vi "testPositiveFixInt.vi"(8 "error in (no error)":errorcluster, 11 "TestCase in":refnum<class "MsgPackSerializerTest.lvclass">) -> (0 "error out":errorcluster, 3 "TestCase out":refnum<class "MsgPackSerializerTest.lvclass">)   [LabVIEW 2015, in "MsgPackSerializerTest.lvclass"]
uses:
  MsgPackSerializerTest.lvclass
  MsgPackSerializer/MsgPackSerializer.lvclass
  <vilib>/addons/_JKI Toolkits/VI Tester/TestCase.llb/TestCase.lvclass
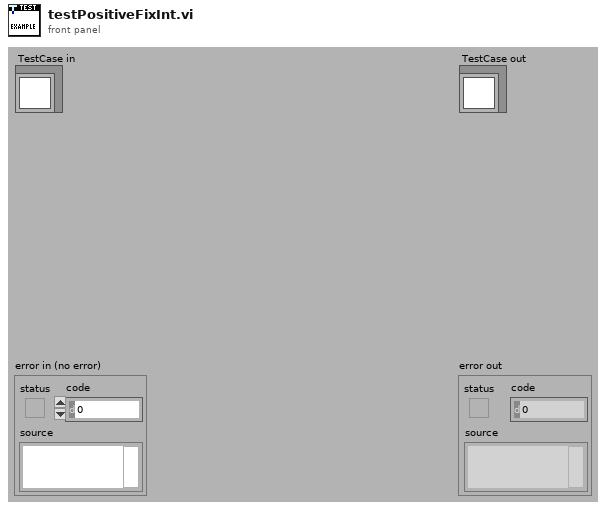
[diagram p1: front panel]
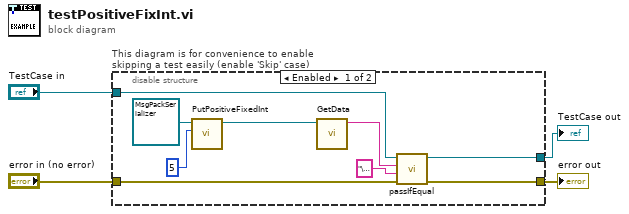
[diagram p0: block diagram]
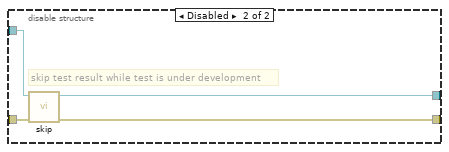
[diagram p2: hidden frame]
diagram:
  n1 = disable-structure "This diagram is for convenience to enable skipping a test easily (enable 'Skip' case)" shown="Enabled" {
    disable-tunnel: "TestCase in" -> [w13 w17]
    disable-tunnel: [w12 w15] -> w1
    disable-tunnel: [w11 w16] -> w3
    disable-tunnel: "error in (no error)" -> [w8 w14]
    frame Enabled {
      n2 = call "PutPositiveFixedInt.vi"("Number"=u8 5, "MsgPackSerializer in"=refnum<class "MsgPackSerializer.lvclass"> refnum ("MsgPackSerializer.lvclass")) -> ("MsgPackSerializer out"=w6:refnum<class "MsgPackSerializer.lvclass">)  [unwired: 8 in, 1 out]
      n3 = call "GetData.vi"("MsgPackSerializer in"=w6) -> ("Data"=w5:string)  [unwired: 9 in, 1 out]
      n4 = call-dynamic "passIfEqual.vi"("error in (no error)"=w8, "y"="\u0005" ("text"), "x"=w5, "TestCase in"=w13) -> ("error out"=w11:errorcluster, "TestCase out"=w12:refnum<class "MsgPackSerializerTest.lvclass">)  [unwired: 6 in]
    }
    frame Disabled {
      # "skip test result while test is under development"
      n5 = call <vilib>:"skip.vi"("error in (no error)"=w14, "TestCase in"=w17) -> ("error out"=w16:errorcluster, "TestCase out"=w15:refnum<class "MsgPackSerializerTest.lvclass">)  [unwired: 8 in]
    }
  }
  "error out" <- w3
  "TestCase out" <- w1
